vi "Rtheta to XY.vi"(2 "theta (deg)":dbl, 3 "R":dbl) -> (0 "Y":dbl, 1 "X":dbl)   [LabVIEW 2012]
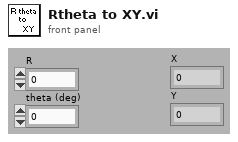
[diagram p1: front panel]
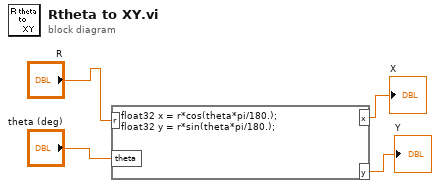
[diagram p0: block diagram]
diagram:
  n1 = formula code="float32 x = r*cos(theta*pi/180.);\nfloat32 y = r*sin(theta*pi/180.);"("r"="R", "theta"="theta (deg)") -> ("x"=→"X":sgl, "y"=→"Y":sgl)
